vi "myRIO_BRig_RT_dataLC_ENL1_Count_NS_l1.vi"() -> (2 "output_ENL1_Count_NS_l1":i32)   [LabVIEW 2014]
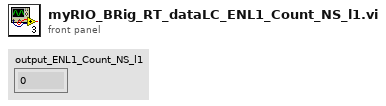
[diagram p1: front panel]
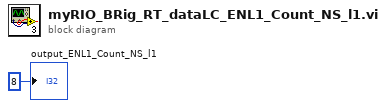
[diagram p0: block diagram]
diagram:
  "output_ENL1_Count_NS_l1" <- 8 ("output_iBlock")
